vi "Configure Date and Time.vi"(8 "error in (no error)":errorcluster, 10 "date and time":timestamp, 11 "VGC in":refnum<class "PL Inficon VGC.lvclass">) -> (0 "error out":errorcluster, 2 "date and time":timestamp, 3 "VGC out":refnum<class "PL Inficon VGC.lvclass">)   [LabVIEW 2015, in "PL Inficon VGC.lvclass"]
doc: "Configures date and time."
uses:
  PL Inficon VGC.lvclass
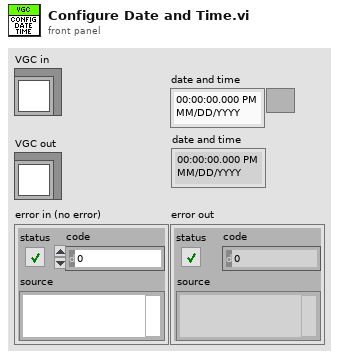
[diagram p1: front panel]
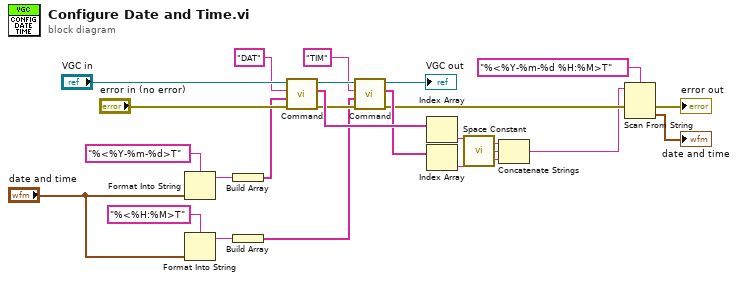
[diagram p0: block diagram]
diagram:
  n1 = Format Into String(format string="%<%Y-%m-%d>T", "date and time") -> (resulting string=w16:string)  [unwired: 2 in, 1 out]
  n2 = Format Into String(format string="%<%H:%M>T", "date and time") -> (resulting string=w15:string)  [unwired: 2 in, 1 out]
  n3 = Build Array(w16) -> (w14:string[])
  n4 = Build Array(w15) -> (w8:string[])
  n5 = call "Command.vi"("error in (no error)"="error in (no error)", "parameters"=w14, "command"="DAT" ("format string"), "VGC in"="VGC in") -> ("error out"=w10:errorcluster, "response data"=w13:string[], "VGC out"=w12:refnum<class "PL Inficon VGC.lvclass">)  [unwired: 5 in]
  n6 = call "Command.vi"("error in (no error)"=w10, "parameters"=w8, "command"="TIM" ("format string"), "VGC in"=w12) -> ("error out"=w3:errorcluster, "response data"=w7:string[], "VGC out"=→"VGC out":refnum<class "PL Inficon VGC.lvclass">)  [unwired: 5 in]
  n7 = Index Array(array=w13) -> (element=w6:string)  [unwired: 1 in]
  n8 = Index Array(array=w7) -> (element=w5:string)  [unwired: 1 in]
  n9 = call <vilib>:"Space Constant.vi"() -> ("String"=w18:string)
  n10 = Concatenate Strings(w6, w18, w5) -> (w1:string)
  n11 = Scan From String(format string="%<%Y-%m-%d %H:%M>T", input string=w1, error in=w3) -> (error out=→"error out":errorcluster, output 1=→"date and time":timestamp)  [unwired: 2 in, 2 out]
